vi "ManualClimb.vi"(10 "CopilotPOV":i16, 11 "CopilotAxes":dbl[](array[numeric])) -> (0 "ActuateBackClimb":dbl, 1 "ActuateFrontClimb":dbl, 2 "DropWheel":bool, 3 "ClimbDrive":bool)   [LabVIEW 2018]
uses:
  Globals.vi
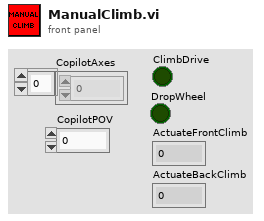
[diagram p1: front panel]
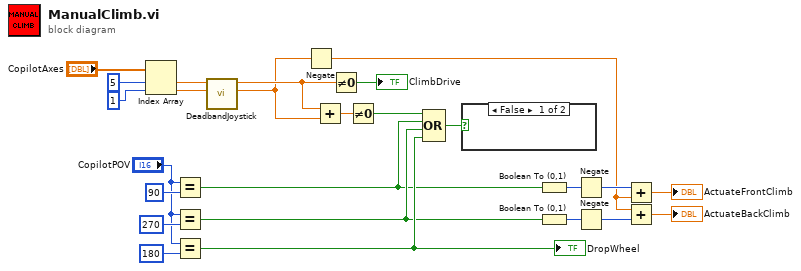
[diagram p0: block diagram]
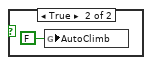
[diagram p2: hidden frame]
diagram:
  n1 = Index Array(array="CopilotAxes", index #1=5 ("index"), index #2=1 ("index")) -> (element #1=w8:dbl, element #2=w7:dbl)
  n2 = Equal?(x="CopilotPOV", y=i16 90) -> (x = y?=w9:bool)
  n3 = Equal?(x="CopilotPOV", y=i16 270) -> (x = y?=w10:bool)
  n4 = Equal?(x="CopilotPOV", y=i16 180) -> (x = y?=w11:bool)
  "DropWheel" <- w11
  n5 = call "DeadbandJoystick.vi"("Y"=w7, "X"=w8) -> ("Y'"=w12:dbl, "X'"=w13:dbl)  [unwired: 7 in, 1 out]
  n6 = Negate(x=w12) -> (-x=w16:dbl)
  n7 = Add(x=w13, y=w12) -> (x+y=w21:dbl)
  n8 = Not Equal To 0?(x=w13) -> (x != 0?=→"ClimbDrive":bool)
  n9 = Not Equal To 0?(x=w21) -> (x != 0?=w14:bool)
  n10 = Compound Arithmetic op=OR(w14, w9, w10, w11) -> (w1:bool)
  n11 = case shown="False" w1 {
    frame False {
    }
    frame True {
      n12 = global write "Globals.vi" "AutoClimb"(FALSE ("AutoClimb")) -> ()
    }
  }
  n13 = Boolean To (0,1)(Boolean=w9) -> (0, 1=w19:i16)
  n14 = Boolean To (0,1)(Boolean=w10) -> (0, 1=w20:i16)
  n15 = Negate(x=w19) -> (-x=w18:i16)
  n16 = Negate(x=w20) -> (-x=w17:i16)
  n17 = Add(x=w18, y=w16) -> (x+y=→"ActuateFrontClimb":dbl)
  n18 = Add(x=w16, y=w17) -> (x+y=→"ActuateBackClimb":dbl)
